vi "Write Board.vi"(8 "error in (no error)":errorcluster, 10 "Board":refnum<class "Board.lvclass">, 11 "Software License Manager in":refnum<class "Software License Manager.lvclass">) -> (0 "error out":errorcluster, 3 "Software License Manager out":refnum<class "Software License Manager.lvclass">)   [LabVIEW 2025, in "SW License Manager.lvlib" / "Software License Manager.lvclass"]
uses:
  Software License Manager.lvclass
  Board/Board.lvclass
  Software License Manager.lvclass/Software License Manager.ctl
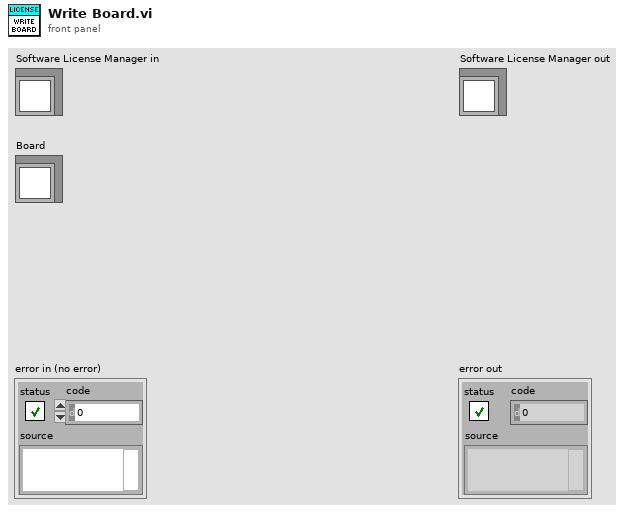
[diagram p1: front panel]
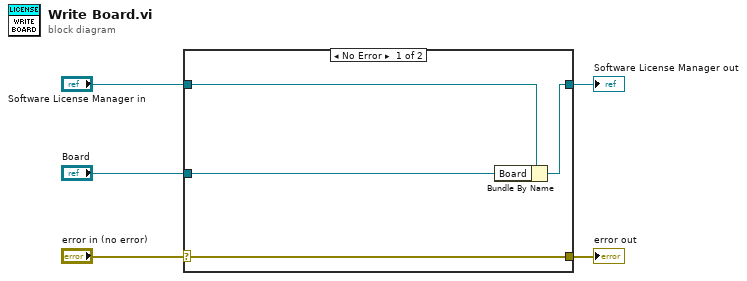
[diagram p0: block diagram]
diagram:
  n1 = case shown="No Error" "error in (no error)" {
    selector: "error in (no error)" -> [w9 w10]
    tunnel: [w9 w10] -> w4
    tunnel: [w7 w11] -> w2
    tunnel: "Software License Manager in" -> [w8 w11]
    tunnel: "Board" -> [w6 _]
    frame No Error {
      n2 = Bundle By Name(cluster=w8, "Board"=w6) -> (w7:refnum<class "Software License Manager.lvclass">)
    }
    frame Error {
    }
  }
  "error out" <- w4
  "Software License Manager out" <- w2
